vi "Rhythm-Plot Pattern.vi"(0 "Graph":refnum<vi>, 5 "Y-axis slider":refnum<vi>, 7 "Values":dbl[](array[numeric]), 9 "Mask":i32[](array[numeric]), 11 "error in (no error)":errorcluster, 12 "Data":T1) -> (15 "error out":errorcluster)   [LabVIEW 2020]
uses:
  Rhythm-Data.ctl
  Utility VIs/Math VIs/LinSpace (x0-dx-npts).vi
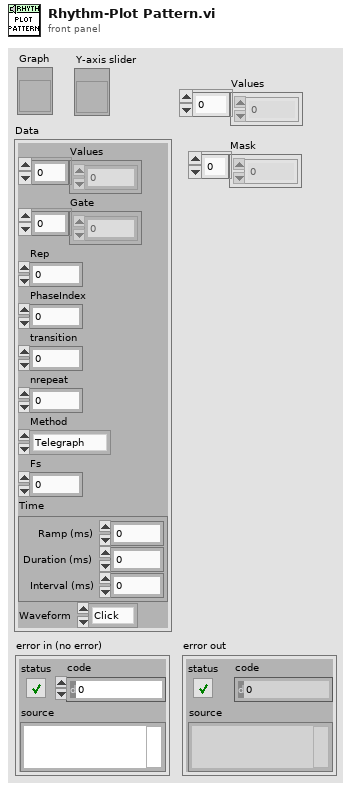
[diagram p1: front panel]
types:
  T1 = typedef "Rhythm-Data.ctl" = cluster{"Values":dbl[], "Gate":dbl[], "Rep":i32, "PhaseIndex":i32, "transition":i32, "nrepeat":i32, "Method":enum16{"Telegraph", "Interval"}, "Fs":dbl, "Time":cluster{"Ramp (ms)":dbl, "Duration (ms)":dbl, "Interval (ms)":dbl}, "Waveform":enum16{"Click", "Noise"}}
  T2 = typedef "LVPoint32TypeDef.ctl" = cluster{"Horizontal":i32, "Vertical":i32}
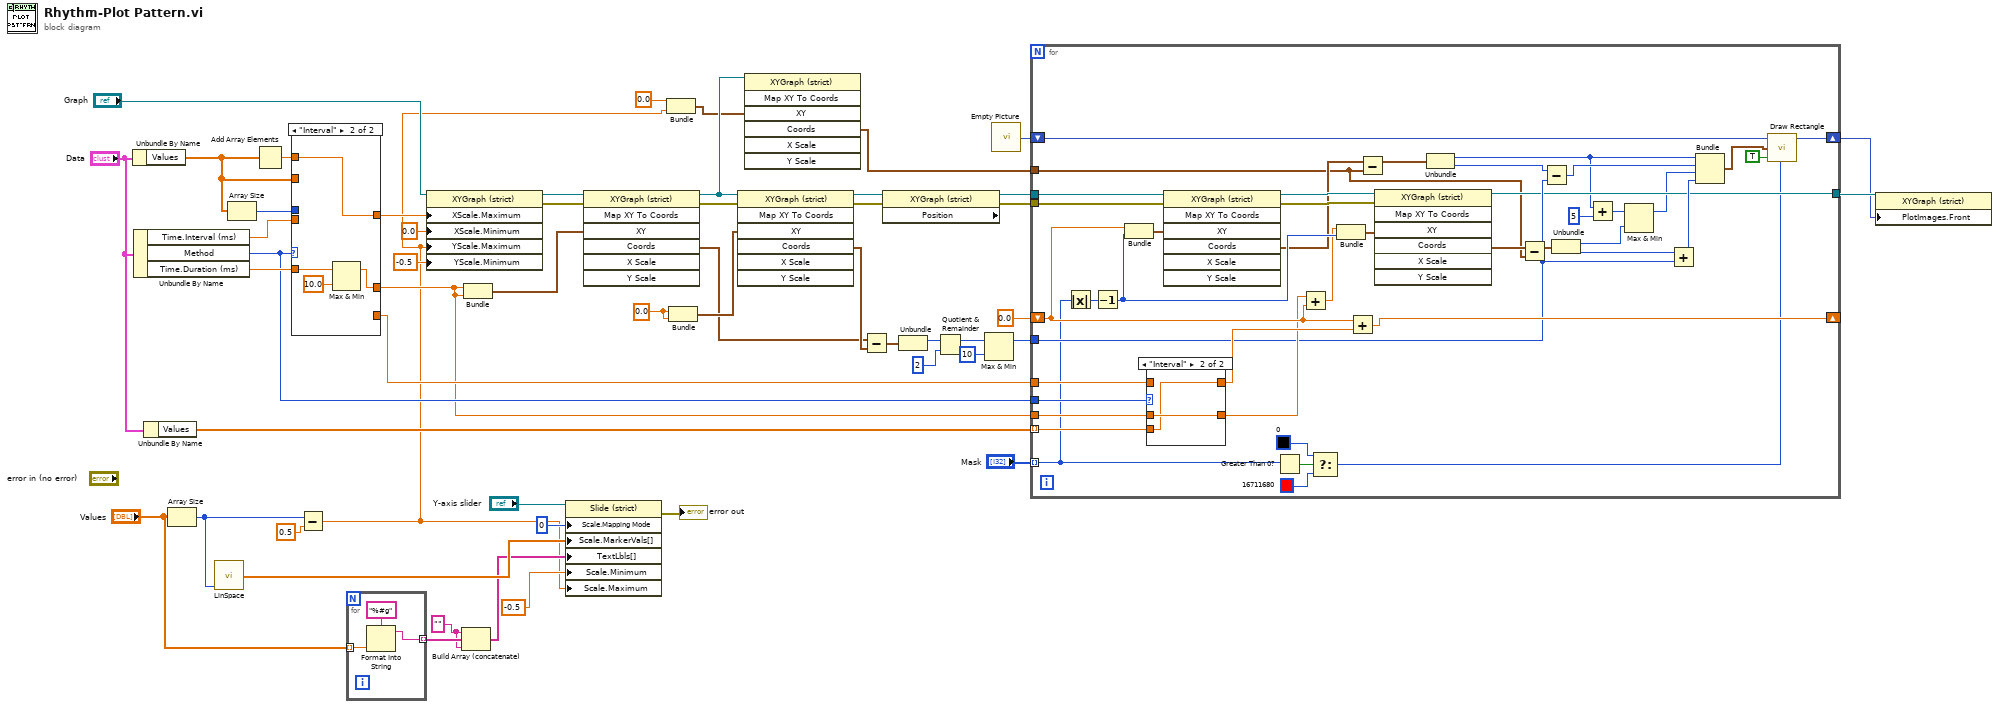
[diagram p0: block diagram]
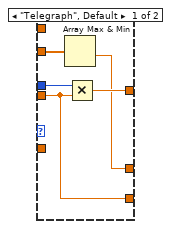
[diagram p3: hidden frame]
diagram:
  w25 = 0.0
  w44 = ""
  n1 = Unbundle By Name("Data") -> ("Values"=w38:dbl[])
  n2 = Unbundle By Name("Data") -> ("Time.Interval (ms)"=w40:dbl, "Method"=w29:enum16{"Telegraph", "Interval"}, "Time.Duration (ms)"=w37:dbl)
  n3 = Unbundle By Name("Data") -> ("Values"=w33:dbl[])
  n4 = Array Size(array="Values") -> (size(s)=w49:i32)
  n5 = call-poly "LinSpace.vi"("npts"=w49) -> ("Array"=w47:dbl[])  [unwired: 3 in, 1 out]
  n6 = Array Size(array=w38) -> (size(s)=w41:i32)
  n7 = Add Array Elements(numeric array=w38) -> (sum=w42:dbl)
  n8 = case shown="\"Interval\"" w29 {
    tunnel: w41 -> [w58 _]
    tunnel: w40 -> [w54 _]
    tunnel: [w57 w62] -> w7
    tunnel: w42 -> [_ w62]
    tunnel: w38 -> [w55 _]
    tunnel: w37 -> [_ w61]
    tunnel: [w56 w59] -> w27
    tunnel: [w54 _] -> w28
    frame "Telegraph", Default {
      n9 = Array Max & Min(array=w55) -> (min value=w56:dbl)  [unwired: 3 out]
      n10 = Multiply(x=w58, y=w54) -> (x*y=w57:dbl)
    }
    frame "Interval" {
      n11 = Max & Min(x=w61, y=10.0) -> (max(x,y)=w59:dbl)  [unwired: 1 out]
    }
  }
  n12 = Subtract(x=w49, y=0.5) -> (x-y=w3:dbl)
  n13 = for {
    tunnel: [w63] -> w50 mode=indexing
    tunnel: "Values" -> [w64] mode=indexing
    n14 = Format Into String(format string="%#g", w64) -> (resulting string=w63:string)  [unwired: 2 in, 1 out]
  }
  n15 = property class="XYGraph (strict)"(reference="Graph", "XScale.Maximum"=w7, "XScale.Minimum"=0.0 ("X Scale.Range:Minimum"), "YScale.Maximum"=w3, "YScale.Minimum"=-0.5 ("Y Scale.Range:Minimum")) -> (reference out=w8:refnum<vi>, error out=w30:errorcluster)  [unwired: 1 in]
  n16 = Build Array (concatenate)(w44, w50, w44) -> (w46:string[])
  n17 = Bundle(w27, w27) -> (w36:cluster{dbl, dbl})  [unwired: 1 in]
  n18 = property class="Slide (strict)"(reference="Y-axis slider", "Scale.Mapping Mode"=u8 0, "Scale.MarkerVals[]"=w47, "TextLbls[]"=w46, "Scale.Minimum"=-0.5 ("Scale.Range:Minimum"), "Scale.Maximum"=w3) -> (error out=→"error out":errorcluster)  [unwired: 1 in, 1 out]
  n19 = invoke class="XYGraph (strict)" method="Map XY To Coords"(reference=w8, error in=w30, "XY"=w36) -> (reference out=w5:refnum<vi>, error out=w31:errorcluster, "Coords"=w23:T2)  [unwired: 4 in, 4 out]
  n20 = Bundle(0.0, w3) -> (w2:cluster{dbl, dbl})  [unwired: 1 in]
  n21 = Bundle(w25, w25) -> (w26:cluster{dbl, dbl})  [unwired: 1 in]
  n22 = invoke class="XYGraph (strict)" method="Map XY To Coords"(reference=w5, error in=w31, "XY"=w26) -> (reference out=w11:refnum<vi>, error out=w14:errorcluster, "Coords"=w24:T2)  [unwired: 4 in, 4 out]
  n23 = invoke class="XYGraph (strict)" method="Map XY To Coords"(reference=w5, "XY"=w2) -> ("Coords"=w1:T2)  [unwired: 5 in, 6 out]
  n24 = Subtract(x=w23, y=w24) -> (x-y=w22:T2)
  n25 = property class="XYGraph (strict)" props=["Position"](reference=w11, error in=w14) -> (reference out=w13:refnum<vi>, error out=w12:errorcluster)  [unwired: 1 out]
  n26 = Unbundle(w22) -> ("Horizontal"=w21:i32)  [unwired: 1 out]
  n27 = Quotient & Remainder(x=w21, y=2) -> (x-y*floor(x/y)=w19:i32)  [unwired: 1 out]
  n28 = Max & Min(x=w19, y=10) -> (max(x,y)=w16:i32)  [unwired: 1 out]
  n29 = call "Empty Picture"() -> ("empty picture"=w6:picture)
  n30 = for {
    tunnel: "Mask" -> [w70] mode=indexing
    tunnel: w33 -> [w97] mode=indexing
    shift-right: [w94] -> _
    shift-left: 0.0 -> [w91]
    shift-right: [w106] -> w17
    shift-left: w6 -> [w107]
    tunnel: w13 -> [w103]
    tunnel: w12 -> [w102]
    tunnel: w29 -> [w98]
    tunnel: w28 -> [w96]
    tunnel: w27 -> [w89]
    tunnel: w16 -> [w82]
    tunnel: [w79] -> w18
    tunnel: w1 -> [w76]
    n31 = Absolute Value(x=w70) -> (abs(x)=w104:i32)
    n32 = Decrement(x=w104) -> (x-1=w93:i32)
    n33 = Bundle(w91, w93) -> (w101:cluster{dbl, i32})  [unwired: 1 in]
    n34 = case shown="\"Interval\"" w98 {
      tunnel: w97 -> [w108 w110]
      tunnel: w96 -> [w109 _]
      tunnel: [w109 w110] -> w95
      tunnel: w89 -> [_ w111]
      tunnel: [w108 w111] -> w88
      frame "Telegraph", Default {
      }
      frame "Interval" {
      }
    }
    n35 = invoke class="XYGraph (strict)" method="Map XY To Coords"(reference=w103, error in=w102, "XY"=w101) -> (reference out=w100:refnum<vi>, error out=w99:errorcluster, "Coords"=w86:T2)  [unwired: 4 in, 4 out]
    n36 = Greater Than 0?(x=w70) -> (x > 0?=w69:bool)
    n37 = Add(x=w88, y=w91) -> (x+y=w90:dbl)
    n38 = Select(t=u32 0, s=w69, f=u32 16711680) -> (s? t:f=w66:u32)
    n39 = Bundle(w90, w93) -> (w92:cluster{dbl, i32})  [unwired: 1 in]
    n40 = Add(x=w91, y=w95) -> (x+y=w94:dbl)
    n41 = Subtract(x=w86, y=w76) -> (x-y=w78:T2)
    n42 = invoke class="XYGraph (strict)" method="Map XY To Coords"(reference=w100, error in=w99, "XY"=w92) -> (reference out=w79:refnum<vi>, "Coords"=w87:T2)  [unwired: 4 in, 5 out]
    n43 = Unbundle(w78) -> ("Horizontal"=w75:i32, "Vertical"=w85:i32)
    n44 = Subtract(x=w87, y=w76) -> (x-y=w77:T2)
    n45 = Subtract(x=w85, y=w82) -> (x-y=w84:i32)
    n46 = Unbundle(w77) -> ("Horizontal"=w72:i32, "Vertical"=w83:i32)
    n47 = Add(x=w75, y=5) -> (x+y=w73:i32)
    n48 = Max & Min(x=w73, y=w72) -> (max(x,y)=w71:i32)  [unwired: 1 out]
    n49 = Add(x=w83, y=w82) -> (x+y=w81:i32)
    n50 = Bundle("Horizontal"=w75, w84, w71, w81) -> (w80:cluster{"Horizontal":i32, i32, i32, i32})  [unwired: 1 in]
    n51 = call <vilib>:"Draw Rectangle.vi"("picture"=w107, "rect"=w80, "fill?(F)"=TRUE, "color(black)"=w66) -> ("new picture"=w106:picture)  [unwired: 5 in]
  }
  n52 = property class="XYGraph (strict)"(reference=w18, "PlotImages.Front"=w17) -> ()  [unwired: 1 in, 2 out]
